vi "SSI_Command.vi"(1 "Opera":u16(ring) items=["Set", "Query"], 2 "Paramter":string, 3 "channel":u16(ring)=1 items=["A"=1, "B"=2, "None"=0], 4 "Command Type":u16(ring) items=["ISRC", "IGND", "ICPL", "ILIN", "PHAS", "FMOD", "RSLP", "FREQ", "SWPT", "SLLM", "SULM", "SSLL", "SSLG", "STLM", "SWRM", "IRNG", "SENS", "RMOD", "OFLT", "OFSL", "SYNC", "DMOD", "HARM", "DARB", "SWVT", "SLVL", "SVLL", "SVUL", "SVSL", "SVSG", "SVTM", "SVRM", "RALL", "SNAP", "OUTP", "OAUX", "COUT", "CAUX", "COFP", "CEXP", "FPOP", "OEXP", "*IDN", "*RST", "OVLD", "INOV", "GNOV", "*PLL", "SSET", "RSET", "AGAN", "APHS", "ARSV", "ASCL", "EQCD", "EQCS", "SPED", "SRAT", "SLEN", "SSLE", "STRG", "SPRM", "STRD", "PAUS", "REST", "SPTS", "TRCA", "TEMP", "RSTU", "INHZ", "DEQU", "SADD", "ARNG", "CSPE", "ISRCD", "IGNDD", "ICPLD", "ILIND", "PHASD", "FMODD", "RSLPD", "FREQD", "SWPTD", "SLLMD", "SULMD", "SSLLD", "SSLGD", "STLMD", "SWRMD", "SENSD", "RMODD", "OFLTD", "OFSLD", "SYNCD", "HARMD", "EQCDD", "EQCSD", "SNAPD", "OUTPD", "SWVTD", "SLVLD", "SVLLD", "SVULD", "SVSLD", "SVSGD", "SVTMD", "SVRMD", "SVDCD", "ARSVD", "AGAND", "APHSD", "ASCLD", "FPOPD", "CAUXD", "OEXPD", "SPEDD", "SRATD", "SLEND", "SSLED", "STRGD", "SPRMD", "STRDD", "PAUSD", "RESTD", "SPTSD", "TRCAD", "*IDND", "*RSTD", "INOVD", "GNOVD", "*PLLD", "SSETD", "RSETD", "RALLD", "NIPA", "NSMA", "NGWA", "NMAC", "NMOD", "TRIG", "TRCB", "INHZD", "ISAMD", "IRAGD", "RRAGD", "SOFFD", "DMODD", "COUTD", "COFPD", "CEXPD", "ARNGD", "OAUXD", "TRIM", "SUITD", "SNHZD", "AOFSD"]) -> (0 "Output string":string)   [LabVIEW 2019]
panel:
  in  "Command":string[](array[string])=["ISRC", "IGND", "ICPL", "ILIN", "PHAS", "FMOD", "RSLP", "FREQ", "SWPT", "SLLM", "SULM", "SSLL", "SSLG", "STLM", "SWRM", "IRNG", "SENS", "RMOD", "OFLT", "OFSL", "SYNC", "DMOD", "HARM", "DARB", "SWVT", "SLVL", "SVLL", "SVUL", "SVSL", "SVSG", "SVTM", "SVRM", "RALL", "SNAP", "OUTP", "OAUX", "COUT", "CAUX", "COFP", "CEXP", "FPOP", "OEXP", "*IDN", "*RST", "OVLD", "INOV", "GNOV", "*PLL", "SSET", "RSET", "AGAN", "APHS", "ARSV", "ASCL", "EQCD", "EQCS", "SPED", "SRAT", "SLEN", "SSLE", "STRG", "SPRM", "STRD", "PAUS", "REST", "SPTS", "TRCA", "TEMP", "RSTU", "INHZ", "DEQU", "SADD", "ARNG", "CSPE", "ISRCD", "IGNDD", "ICPLD", "ILIND", "PHASD", "FMODD", "RSLPD", "FREQD", "SWPTD", "SLLMD", "SULMD", "SSLLD", "SSLGD", "STLMD", "SWRMD", "SENSD", "RMODD", "OFLTD", "OFSLD", "SYNCD", "HARMD", "EQCDD", "EQCSD", "SNAPD", "OUTPD", "SWVTD", "SLVLD", "SVLLD", "SVULD", "SVSLD", "SVSGD", "SVTMD", "SVRMD", "SVDCD", "ARSVD", "AGAND", "APHSD", "ASCLD", "FPOPD", "CAUXD", "OEXPD", "SPEDD", "SRATD", "SLEND", "SSLED", "STRGD", "SPRMD", "STRDD", "PAUSD", "RESTD", "SPTSD", "TRCAD", "*IDND", "*RSTD", "INOVD", "GNOVD", "*PLLD", "SSETD", "RSETD", "RALLD", "NIPA", "NSMA", "NGWA", "NMAC", "NMOD", "TRIG", "TRCB", "INHZD", "ISAMD", "IRAGD", "RRAGD", "SOFFD", "DMODD", "COUTD", "COFPD", "CEXPD", "ARNGD", "OAUXD", "TRIM"]
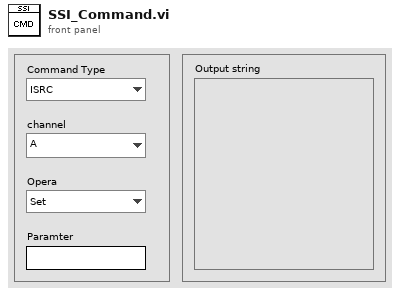
[diagram p1: front panel]
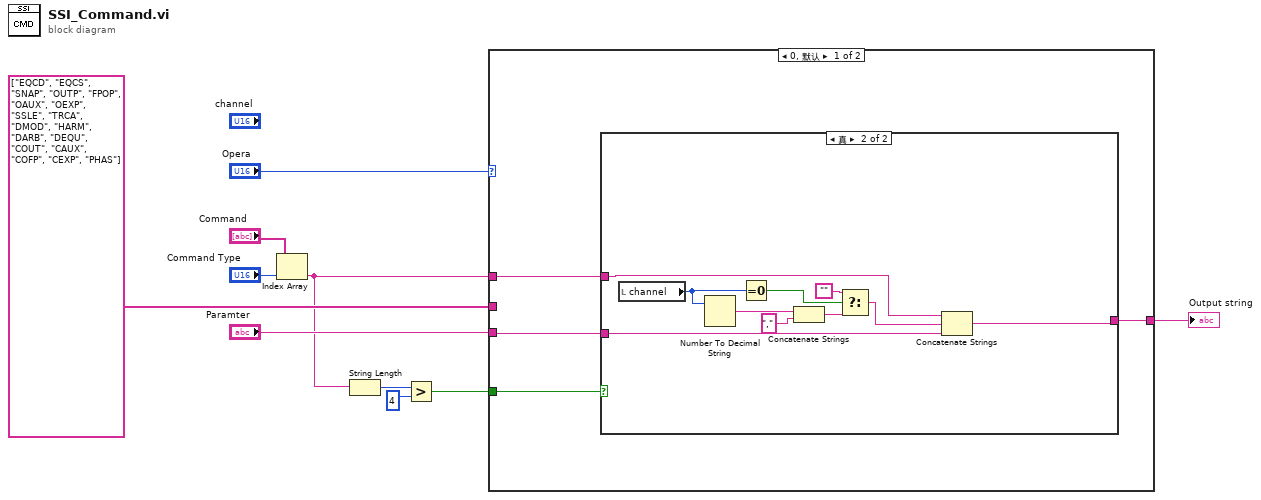
[diagram p0: block diagram]
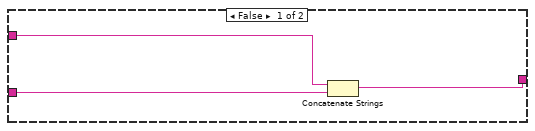
[diagram p2: hidden frame]
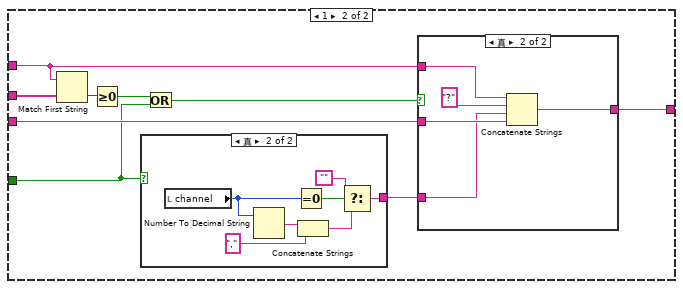
[diagram p3: hidden frame]
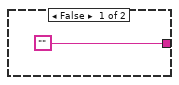
[diagram p4: hidden frame]
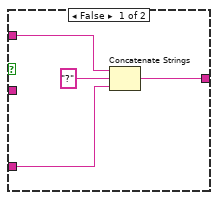
[diagram p5: hidden frame]
diagram:
  n1 = Index Array(array="Command", index="Command Type") -> (element=w3:string)
  n2 = String Length(string=w3) -> (length=w7:i32)
  n3 = Greater?(x=w7, y=4) -> (0:w8:bool)
  n4 = case shown="0, 默认" "Opera" {
    tunnel: [w14 w36] -> w2
    tunnel: w3 -> [w13 w32]
    tunnel: "Paramter" -> [w11 w35]
    tunnel: string[] ["EQCD", "EQCS", "SNAP", "OUTP", "FPOP", "OAUX", "OEXP", "SSLE", "TRCA", "DMOD", "HARM", "DARB", "DEQU", "COUT", "CAUX", "COFP", "CEXP", "PHAS"] ("字符串数组") -> [_ w33]
    tunnel: w8 -> [w12 w29]
    frame 0, Default {
      n5 = case shown="真" w12 {
        tunnel: [w17 w27] -> w14
        tunnel: w13 -> [w16 w26]
        tunnel: w11 -> [w15 w25]
        frame False {
          n6 = Concatenate Strings(w16, w15) -> (w17:string)
        }
        frame True {
          n7 = local read "channel"() -> (w22:u16)
          n8 = Number To Decimal String(number=w22) -> (decimal integer string=w19:string)  [unwired: 1 in]
          n9 = Equal To 0?(x=w22) -> (x = 0?=w24:bool)
          n10 = Concatenate Strings(w19, "," ("字符串")) -> (w20:string)
          n11 = Select(t="", s=w24, f=w20) -> (s? t:f=w21:string)
          n12 = Concatenate Strings(w26, w21, w25) -> (w27:string)
        }
      }
    }
    frame 1 {
      n13 = Match First String(2:w33, 3:w32) -> (0:w34:i32)  [unwired: 1 out]
      n14 = Greater Or Equal To 0?(x=w34) -> (x >= 0?=w30:bool)
      n15 = case shown="真" w29 {
        tunnel: ["" w41] -> w28
        frame False {
        }
        frame True {
          n16 = local read "channel"() -> (w39:u16)
          n17 = Number To Decimal String(number=w39) -> (decimal integer string=w44:string)  [unwired: 1 in]
          n18 = Equal To 0?(x=w39) -> (x = 0?=w38:bool)
          n19 = Concatenate Strings(w44, "," ("字符串")) -> (w42:string)
          n20 = Select(t="", s=w38, f=w42) -> (s? t:f=w41:string)
        }
      }
      n21 = Or(x=w30, y=w29) -> (x .or. y?=w31:bool)
      n22 = case shown="真" w31 {
        tunnel: [w48 w53] -> w36
        tunnel: w32 -> [w47 w51]
        tunnel: w35 -> [_ w52]
        tunnel: w28 -> [w45 w49]
        frame False {
          n23 = Concatenate Strings(w47, "?" ("字符串"), w45) -> (w48:string)
        }
        frame True {
          n24 = Concatenate Strings(w51, "?" ("字符串"), w49, w52) -> (w53:string)
        }
      }
    }
  }
  "Output string" <- w2
